vi "Dequeue Error.vi"(8 "error in (no error)":errorcluster) -> (0 "error out":errorcluster, 1 "Variant":variant, 2 "String":string, 3 "Queue Out":T1)   [LabVIEW 2023, in "Error Handling.lvlib"]
uses:
  Error Handling.lvlib
  Internal Communication/Controls/Queue.ctl
  Internal Communication/Internal Communication.lvlib
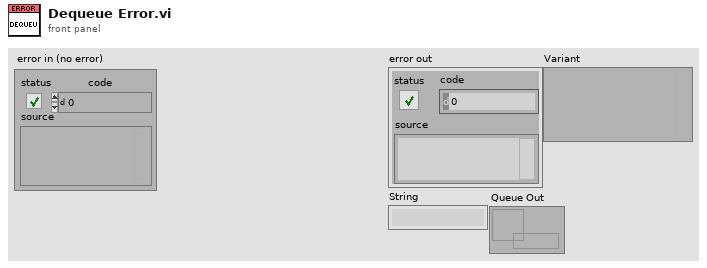
[diagram p1: front panel]
types:
  T1 = typedef "Queue.ctl" = refnum<queue>
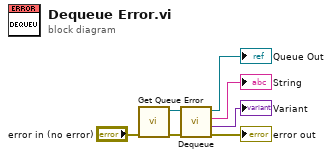
[diagram p0: block diagram]
diagram:
  n1 = call "Get Queue Error.vi"("error in (no error)"="error in (no error)") -> ("error out"=w3:errorcluster, "Error Queue"=w2:refnum<queue>)  [unwired: 9 in]
  n2 = call "Dequeue.vi"("error in (no error)"=w3, "Queue In"=w2) -> ("error out"=→"error out":errorcluster, "Variant"=→"Variant":variant, "String"=→"String":string, "Queue Out"=→"Queue Out":T1)  [unwired: 6 in]
